vi "GetName.vi"(8 "error in (no error)":errorcluster, 11 "3D Object in":refnum<class "3D Object.lvclass">) -> (0 "error out":errorcluster, 2 "Name":string, 3 "3D Object out":refnum<class "3D Object.lvclass">)   [LabVIEW 2015, in "3D Object.lvclass"]
uses:
  3D Object.lvclass
  3D Object.lvclass/3D Object.ctl
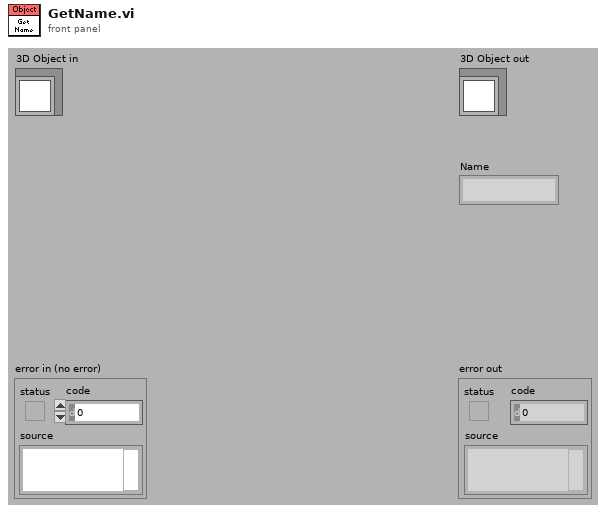
[diagram p1: front panel]
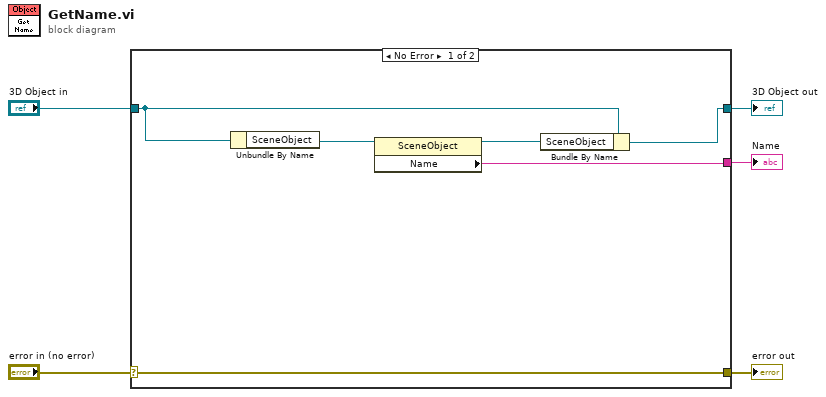
[diagram p0: block diagram]
diagram:
  n1 = case shown="No Error" "error in (no error)" {
    selector: "error in (no error)" -> [w11 w13]
    tunnel: [w11 w13] -> w4
    tunnel: [w7 w12] -> w2
    tunnel: "3D Object in" -> [w8 w12]
    tunnel: [w6 _] -> w1
    frame No Error {
      n2 = Unbundle By Name(w8) -> ("SceneObject"=w10:refnum<vi>)
      n3 = property class="SceneObject"(reference=w10) -> (reference out=w9:refnum<vi>, "Name"=w6:string)  [unwired: 1 in, 1 out]
      n4 = Bundle By Name(cluster=w8, "SceneObject"=w9) -> (w7:refnum<class "3D Object.lvclass">)
    }
    frame Error {
    }
  }
  "error out" <- w4
  "3D Object out" <- w2
  "Name" <- w1
